vi "BuildHWI.vi"(8 "error in (no error)":errorcluster, 10 "Master Device in":refnum<class "Master Device.lvclass">, 11 "Aerotech_Soloist in":refnum<class "Aerotech_Soloist.lvclass">) -> (0 "error out":errorcluster, 2 "Master Device out":refnum<class "Master Device.lvclass">, 3 "Aerotech_Soloist out":refnum<class "Aerotech_Soloist.lvclass">)   [LabVIEW 2013, in "Aerotech_Soloist.lvclass"]
doc: "The previous subVI Prune.vi took the \"prepared\" private data and removed unnecessary points. Here in BuildHWI, one should turn the \"prepared\" data into a HWI that can be programmed to the physical device.\n (1) Flatten the data structure and put in normal time order"
uses:
  Aerotech_Soloist.lvclass
  Master Device/Master Device.lvclass
  Aerotech_Soloist.lvclass/Aerotech_Soloist.ctl
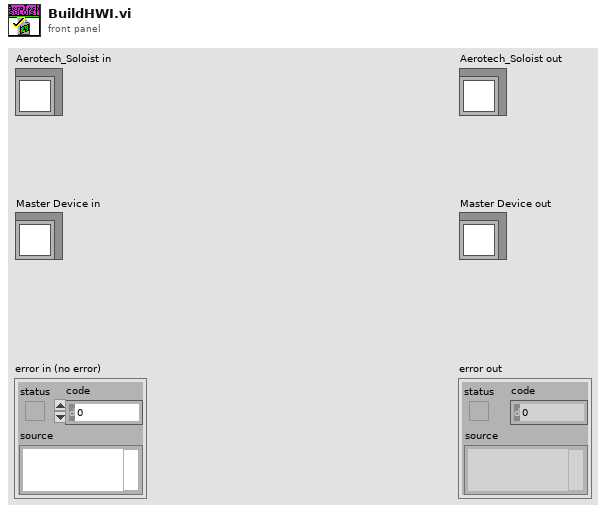
[diagram p1: front panel]
types:
  T1 = typedef "Aerotech_Soloist.lvclass/ParsedSWILine.ctl" = cluster{"ParameterScript":string, "CommandScript":string}
  T2 = typedef "SlaveInfo.ctl" = cluster{"Triggering":bool[][], "Ramp Info":T3[], "Line Inversion":bool[], "Slaved Digital Channels":cluster{"Master Channel Number":i32, "Output States":bool[]}[]}
  T3 = typedef "RampInfo.ctl" = cluster{"Table Ramp Index":i32, "Ramp Time":dbl, "Number of Steps":i32, "Instruction Array Index":i32}
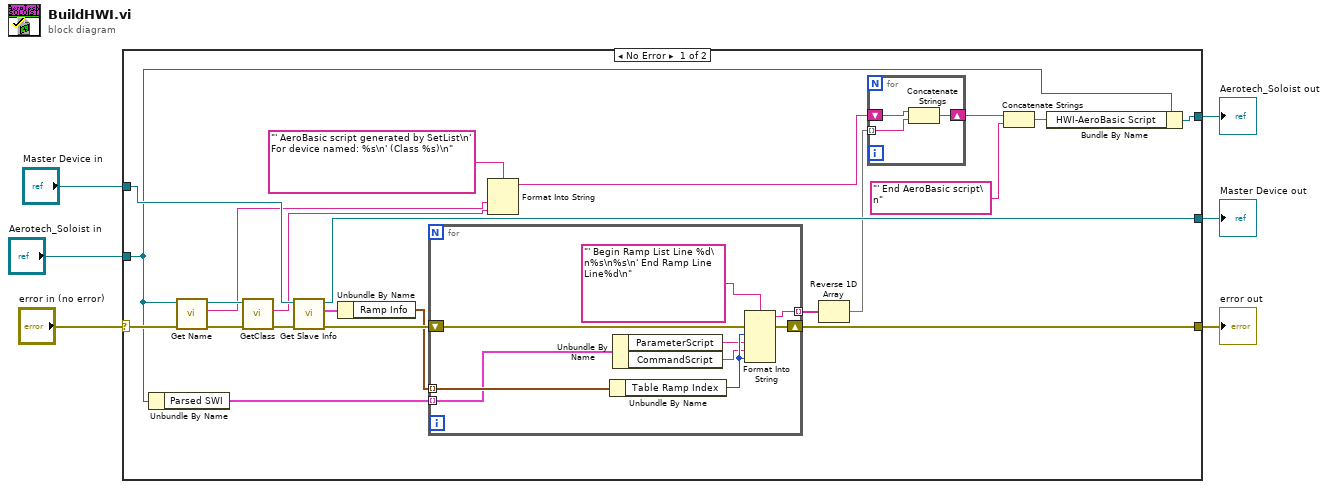
[diagram p0: block diagram]
diagram:
  n1 = case shown="No Error" "error in (no error)" {
    selector: "error in (no error)" -> [w21 w43]
    tunnel: "Aerotech_Soloist in" -> [w12 w41]
    tunnel: "Master Device in" -> [w28 w42]
    tunnel: [w7 w43] -> w3
    tunnel: [w26 w42] -> w2
    tunnel: [w11 w41] -> w1
    frame No Error {
      n2 = Unbundle By Name(w12) -> ("Parsed SWI"=w27:T1[])
      n3 = call-dynamic "Get Name.vi"("error in (no error)"=w21, "Device in"=w12) -> ("error out"=w22:errorcluster, "Name"=w19:string, "Device out"=w23:refnum<class "Aerotech_Soloist.lvclass">)  [unwired: 7 in]
      n4 = call-dynamic "GetClass.vi"("error in (no error)"=w22, "Device in"=w23) -> ("error out"=w20:errorcluster, "Device Class"=w18:string)  [unwired: 7 in, 1 out]
      n5 = call-dynamic "Get Slave Info.vi"("error in (no error)"=w20, "Master Device in"=w28) -> ("error out"=w25:errorcluster, "Slave Info"=w17:T2, "Master Device out"=w26:refnum<class "Master Device.lvclass">)  [unwired: 7 in]
      n6 = Unbundle By Name(w17) -> ("Ramp Info"=w16:T3[])
      n7 = for {
        tunnel: w27 -> [w36] mode=indexing
        shift-right: [w32] -> w7
        shift-left: w25 -> [w33]
        tunnel: w16 -> [w40] mode=indexing
        tunnel: [w38] -> w15 mode=indexing
        n8 = Unbundle By Name(w40) -> ("Table Ramp Index"=w37:i32)
        n9 = Unbundle By Name(w36) -> ("ParameterScript"=w35:string, "CommandScript"=w34:string)
        n10 = Format Into String(format string="' Begin Ramp List Line %d\n%s\n%s\n' End Ramp Line Line%d\n", error in=w33, w37, w35, w34, w37) -> (resulting string=w38:string, error out=w32:errorcluster)  [unwired: 1 in]
      }
      n11 = Format Into String(format string="' AeroBasic script generated by SetList\n' For device named: %s\n' (Class %s)\n", w19, w18) -> (resulting string=w14:string)  [unwired: 2 in, 1 out]
      n12 = Reverse 1D Array(array=w15) -> (reversed array=w13:string[])
      n13 = for {
        shift-right: [w31] -> w10
        shift-left: w14 -> [w30]
        tunnel: w13 -> [w29] mode=indexing
        n14 = Concatenate Strings(w30, w29) -> (w31:string)
      }
      n15 = Concatenate Strings(w10, "' End AeroBasic script\n" ("string")) -> (w8:string)
      n16 = Bundle By Name(cluster=w12, "HWI-AeroBasic Script"=w8) -> (w11:refnum<class "Aerotech_Soloist.lvclass">)
    }
    frame Error {
    }
  }
  "error out" <- w3
  "Aerotech_Soloist out" <- w1
  "Master Device out" <- w2
